vi "calculate_change.vi"(0 "User_cash":T1, 5 "Machine_cash":T1, 7 "Amount":i32 min=0, 11 "error in (no error)":errorcluster) -> (4 "Change_cash":T1, 6 "Machine_cash":T1, 8 "Has_change":bool, 15 "error in (no error) 2":errorcluster)   [LabVIEW 2023, in "Vending_machine.lvlib"]
doc: "Find the change to be returned to the user."
uses:
  Vending_machine.lvlib
  Controls/Cash.ctl
  Controls/change_data.ctl
  Controls/Denominations.ctl
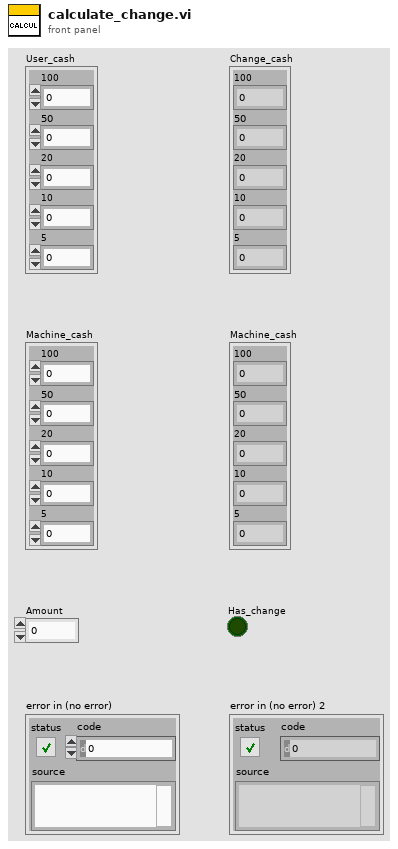
[diagram p1: front panel]
types:
  T1 = typedef "Vending_machine.lvlib/Cash.ctl" = cluster{"100":i32, "50":i32, "20":i32, "10":i32, "5":i32}
  T2 = typedef "Vending_machine.lvlib/change_data.ctl" = cluster{"Change_cash":T1, "Machine_cash":T1, "Change":i32, "Has_change":bool}
  T3 = typedef "Vending_machine.lvlib/Denominations.ctl" = string[]
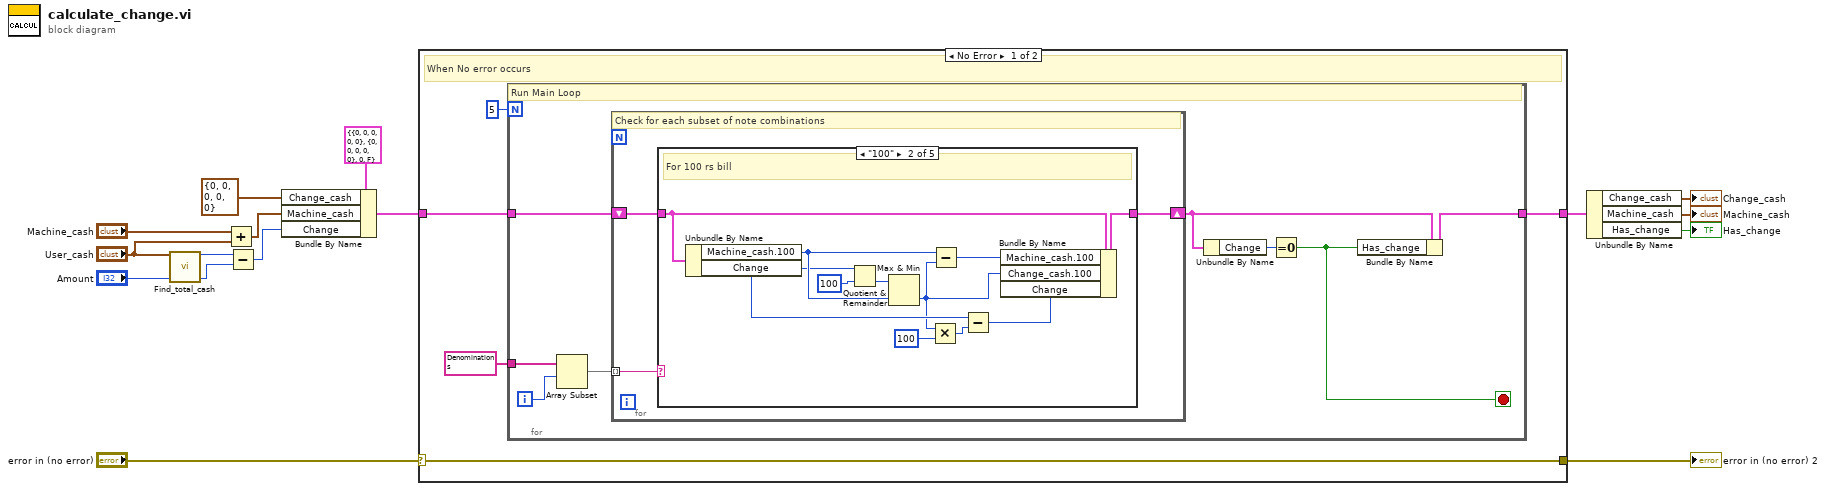
[diagram p0: block diagram]
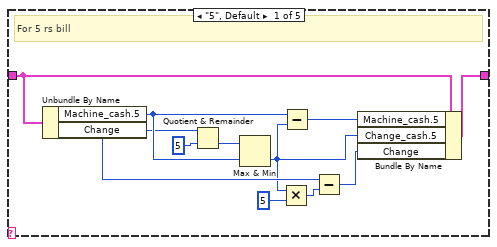
[diagram p2: hidden frame]
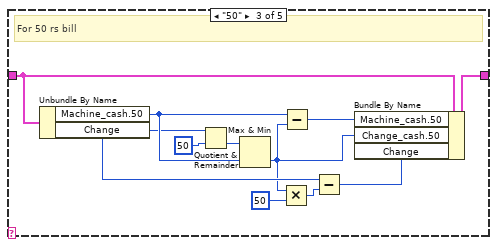
[diagram p3: hidden frame]
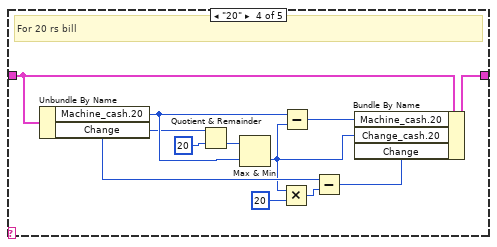
[diagram p4: hidden frame]
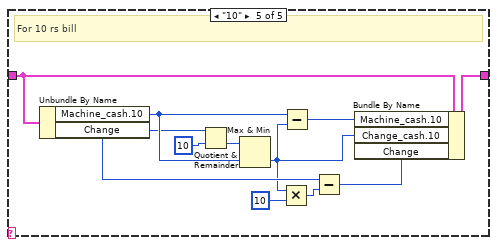
[diagram p5: hidden frame]
diagram:
  n1 = call "Find_total_cash.vi"("Cash"="User_cash") -> ("Total_Cash"=w15:i32)  [unwired: 14 in]
  n2 = Add(x="Machine_cash", y="User_cash") -> (x+y=w10:T1)
  n3 = Subtract(x=w15, y="Amount") -> (x-y=w9:i32)
  n4 = Bundle By Name(cluster=T2 {"Change_cash"={"100"=0, "50"=0, "20"=0, "10"=0, "5"=0}, "Machine_cash"={"100"=0, "50"=0, "20"=0, "10"=0, "5"=0}, "Change"=0, "Has_change"=FALSE}, "Change_cash"=T1 {"100"=0, "50"=0, "20"=0, "10"=0, "5"=0}, "Machine_cash"=w10, "Change"=w9) -> (w7:T2)
  n5 = case shown="No Error" "error in (no error)" {
    selector: "error in (no error)" -> [w16 w88]
    tunnel: w7 -> [w18 w87]
    tunnel: [w17 w87] -> w6
    tunnel: [w16 w88] -> w1
    frame No Error {
      # "When No error occurs"
      n6 = for {
        N: 5 -> [_]
        tunnel: T3 ["100", "50", "20", "10", "5"] ("Array") -> [w28]
        tunnel: w18 -> [w25]
        tunnel: [w22] -> w17
        i -> [w27]
        stop <- w21 stop-if-true
        # "Run Main Loop"
        n7 = Array Subset(array=w28, index=w27) -> (w26:T3)  [unwired: 1 in]
        n8 = for {
          tunnel: w26 -> [w31] mode=indexing
          shift-right: [w29] -> w24
          shift-left: w25 -> [w30]
          # "Check for each subset of note combinations"
          n9 = case shown="\"100\"" w31 {
            tunnel: w30 -> [w40 w51 w62 w73 w84]
            tunnel: [w39 w50 w61 w72 w83] -> w29
            frame "5", Default {
              # "For 5 rs bill"
              n10 = Unbundle By Name(w40) -> ("Machine_cash.5"=w38:i32, "Change"=w35:i32)
              n11 = Quotient & Remainder(x=w35, y=5) -> (floor(x/y)=w41:i32)  [unwired: 1 out]
              n12 = Max & Min(x=w41, y=w38) -> (min(x,y)=w32:i32)  [unwired: 1 out]
              n13 = Multiply(x=w32, y=5) -> (x*y=w34:i32)
              n14 = Subtract(x=w38, y=w32) -> (x-y=w37:i32)
              n15 = Subtract(x=w35, y=w34) -> (x-y=w36:i32)
              n16 = Bundle By Name(cluster=w40, "Machine_cash.5"=w37, "Change_cash.5"=w32, "Change"=w36) -> (w39:T2)
            }
            frame "100" {
              # "For 100 rs bill"
              n17 = Unbundle By Name(w51) -> ("Machine_cash.100"=w49:i32, "Change"=w46:i32)
              n18 = Quotient & Remainder(x=w46, y=100) -> (floor(x/y)=w52:i32)  [unwired: 1 out]
              n19 = Max & Min(x=w52, y=w49) -> (min(x,y)=w43:i32)  [unwired: 1 out]
              n20 = Multiply(x=w43, y=100) -> (x*y=w45:i32)
              n21 = Subtract(x=w49, y=w43) -> (x-y=w48:i32)
              n22 = Subtract(x=w46, y=w45) -> (x-y=w47:i32)
              n23 = Bundle By Name(cluster=w51, "Machine_cash.100"=w48, "Change_cash.100"=w43, "Change"=w47) -> (w50:T2)
            }
            frame "50" {
              # "For 50 rs bill"
              n24 = Unbundle By Name(w62) -> ("Machine_cash.50"=w60:i32, "Change"=w57:i32)
              n25 = Quotient & Remainder(x=w57, y=50) -> (floor(x/y)=w63:i32)  [unwired: 1 out]
              n26 = Max & Min(x=w63, y=w60) -> (min(x,y)=w54:i32)  [unwired: 1 out]
              n27 = Multiply(x=w54, y=50) -> (x*y=w56:i32)
              n28 = Subtract(x=w60, y=w54) -> (x-y=w59:i32)
              n29 = Subtract(x=w57, y=w56) -> (x-y=w58:i32)
              n30 = Bundle By Name(cluster=w62, "Machine_cash.50"=w59, "Change_cash.50"=w54, "Change"=w58) -> (w61:T2)
            }
            frame "20" {
              # "For 20 rs bill"
              n31 = Unbundle By Name(w73) -> ("Machine_cash.20"=w71:i32, "Change"=w68:i32)
              n32 = Quotient & Remainder(x=w68, y=20) -> (floor(x/y)=w74:i32)  [unwired: 1 out]
              n33 = Max & Min(x=w74, y=w71) -> (min(x,y)=w65:i32)  [unwired: 1 out]
              n34 = Multiply(x=w65, y=20) -> (x*y=w67:i32)
              n35 = Subtract(x=w71, y=w65) -> (x-y=w70:i32)
              n36 = Subtract(x=w68, y=w67) -> (x-y=w69:i32)
              n37 = Bundle By Name(cluster=w73, "Machine_cash.20"=w70, "Change_cash.20"=w65, "Change"=w69) -> (w72:T2)
            }
            frame "10" {
              # "For 10 rs bill"
              n38 = Unbundle By Name(w84) -> ("Machine_cash.10"=w82:i32, "Change"=w79:i32)
              n39 = Quotient & Remainder(x=w79, y=10) -> (floor(x/y)=w85:i32)  [unwired: 1 out]
              n40 = Max & Min(x=w85, y=w82) -> (min(x,y)=w76:i32)  [unwired: 1 out]
              n41 = Multiply(x=w76, y=10) -> (x*y=w78:i32)
              n42 = Subtract(x=w82, y=w76) -> (x-y=w81:i32)
              n43 = Subtract(x=w79, y=w78) -> (x-y=w80:i32)
              n44 = Bundle By Name(cluster=w84, "Machine_cash.10"=w81, "Change_cash.10"=w76, "Change"=w80) -> (w83:T2)
            }
          }
        }
        n45 = Unbundle By Name(w24) -> ("Change"=w23:i32)
        n46 = Equal To 0?(x=w23) -> (x = 0?=w21:bool)
        n47 = Bundle By Name(cluster=w24, "Has_change"=w21) -> (w22:T2)
      }
    }
    frame Error {
      # "When an error occurs"
    }
  }
  "error in (no error) 2" <- w1
  n48 = Unbundle By Name(w6) -> ("Change_cash"=→"Change_cash":T1, "Machine_cash"=→"Machine_cash":T1, "Has_change"=→"Has_change":bool)
